vi "LV SciSDK FFT.vi"(7 "FFT Handle In":cluster{"FFT Path":string, "FFT Name":string}, 9 "Board Handle In":T1, 11 "error in (no error)":errorcluster) -> (4 "NI Error Code":i32, 6 "FFT Buffer Out":T2, 8 "FFT Handle Out":cluster{"FFT Path":string, "FFT Name":string}, 10 "Board Handle Out":T1, 15 "error out":errorcluster)   [LabVIEW 2021, in "SciSDK_Labview.lvlib"]
uses:
  SciSDK_Labview.lvlib
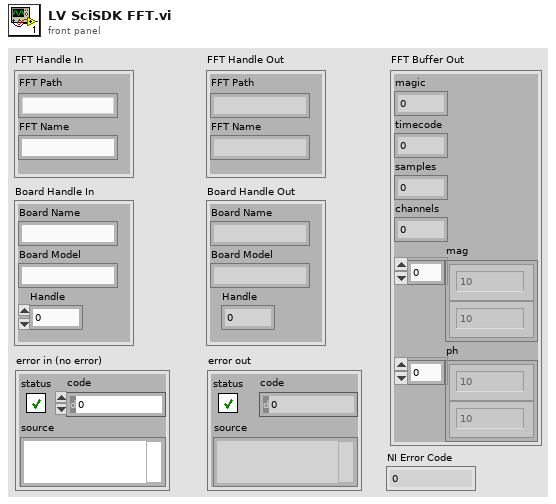
[diagram p1: front panel]
types:
  T1 = cluster{"Board Name":string, "Board Model":string, "Handle":u64}
  T2 = cluster{"magic":u32, "timecode":u32, "samples":u32, "channels":u32, "mag":dbl[], "ph":dbl[]}
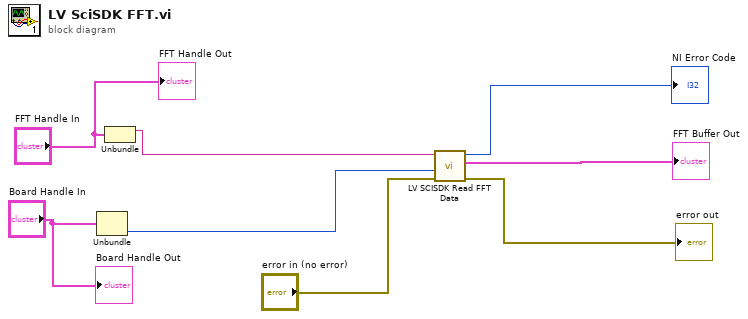
[diagram p0: block diagram]
diagram:
  n1 = Unbundle("Board Handle In") -> ("Handle"=w1:u64)  [unwired: 2 out]
  n2 = Unbundle("FFT Handle In") -> ("FFT Path"=w3:string)  [unwired: 1 out]
  n3 = call "LV SCISDK Read FFT Data.vi"("Path"=w3, "handle"=w1, "error in (no error)"="error in (no error)") -> ("function return"=→"NI Error Code":i32, "buffer out"=→"FFT Buffer Out":T2, "error out"=→"error out":errorcluster)  [unwired: 4 in, 1 out]
  "FFT Handle Out" <- "FFT Handle In"
  "Board Handle Out" <- "Board Handle In"
